vi "Library.Open.vi"(8 "error in (no error)":errorcluster, 10 "Library Path":path, 11 "application reference (local)":refnum<vi>) -> (0 "error out":errorcluster, 3 "Library Reference":refnum<vi>)   [LabVIEW 2011]
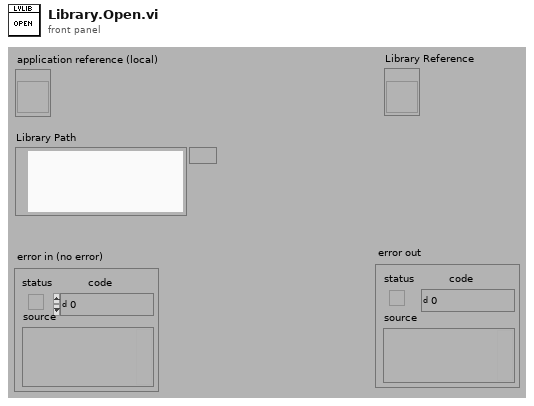
[diagram p1: front panel]
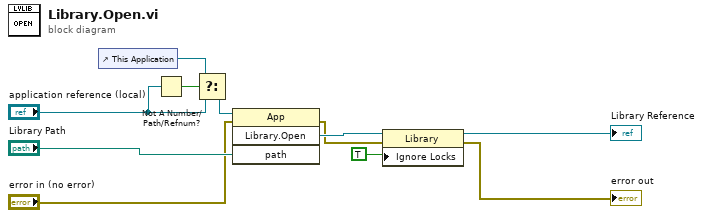
[diagram p0: block diagram]
diagram:
  n1 = control-ref of="This Application"() -> (w8:refnum<vi>)
  n2 = Not A Number/Path/Refnum?(number/path/refnum="application reference (local)") -> (NaN/Path/Refnum?=w9:bool)
  n3 = Select(t=w8, s=w9, f="application reference (local)") -> (s? t:f=w6:refnum<vi>)
  n4 = invoke class="App" method="Library.Open"(reference=w6, error in="error in (no error)", "path"="Library Path") -> (error out=w3:errorcluster, "Open Library"=w4:refnum<vi>)  [unwired: 1 in, 2 out]
  n5 = property class="Library"(reference=w4, error in=w3, "Ignore Locks"=TRUE) -> (reference out=→"Library Reference":refnum<vi>, error out=→"error out":errorcluster)
